vi "Actor1_GUI_N_4.0.0_Main.vi"() -> ()   [LabVIEW 2016, in "Actor1_GUI_N_4.0.0.lvlib"]
uses:
  <resource>/Framework/Providers/Open_GDS/ClassProviders/ActorFramework/4.0.0/Actor1_GUI_N_4.0.0/Actor1_GUI_N_4.0.0.lvlib
  <resource>/Framework/Providers/Open_GDS/ClassProviders/ActorFramework/4.0.0/Actor1_GUI_N_4.0.0/Actor1_GUI_N_4.0.0_class/Actor1_GUI_N_4.0.0.lvclass
  C:/Program Files (x86)/National Instruments/LabVIEW 2016/vi.lib/ActorFramework/Actor/Actor.lvclass
  <vilib>/ActorFramework/Message Enqueuer/Message Enqueuer.lvclass/Message Enqueuer.ctl
  <vilib>/ActorFramework/Message Enqueuer/Enqueue.vi
  <vilib>/ActorFramework/Stop Msg/Stop Msg.lvclass
  C:/Program Files (x86)/National Instruments/LabVIEW 2016/vi.lib/ActorFramework/Message/Message.lvclass
  <vilib>/ActorFramework/Message Priority Queue/Priority Enqueue.vi
  <resource>/Framework/Providers/Open_GDS/ClassProviders/ActorFramework/4.0.0/Actor1_GUI_N_4.0.0/Messages/StartMeasurement_Msg/StartMeasurement_Msg.lvclass
  <vilib>/ActorFramework/Actor/Actor.lvclass
panel:
  in  "Quit":bool
  in  "Start":bool
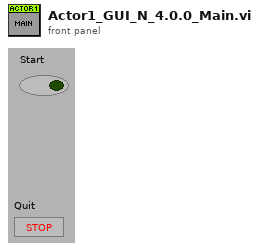
[diagram p1: front panel]
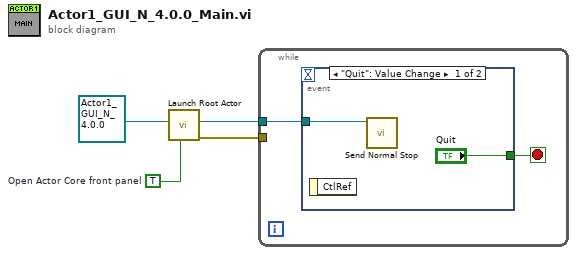
[diagram p0: block diagram]
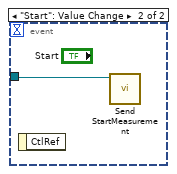
[diagram p2: hidden frame]
diagram:
  w3 = TRUE  # Open Actor Core front panel
  n1 = call <vilib>:"Launch Root Actor.vi"("Open Actor Core front panel? (F)"=w3, "Actor"=refnum<class "Actor1_GUI_N_4.0.0.lvclass"> refnum ("Actor1_GUI_4.0.0.lvlib:Actor1_GUI")) -> ("error out"=w1:errorcluster, "Actor's Enqueuer"=w2:refnum<class "Message Enqueuer.lvclass">)  [unwired: 8 in]
  n2 = while {
    tunnel: w2 -> [w5]
    tunnel: w1 -> [_]
    stop <- w6 stop-if-true
    n3 = event shown="[0] \"Quit\": Value Change" {
      selector: _ -> [_ _]
      dyn-events: _ -> [_ _]
      timeout: _ -> [_ _]
      tunnel: ["Quit" _] -> w6
      tunnel: w5 -> [w7 w9]
      event "Quit": Value Change {
        n4 = event-data() -> ()  [unwired: 1 in, 1 out]
        n5 = call <vilib>:"Send Normal Stop.vi"("Message Enqueuer"=w7) -> ()  [unwired: 10 in, 1 out]
      }
      event "Start": Value Change {
        n6 = event-data() -> ()  [unwired: 1 in, 1 out]
        n7 = call <resource>:"Send StartMeasurement.vi"("Message Enqueuer"=w9) -> ()  [unwired: 10 in, 1 out]
      }
    }
  }
